vi "create_scan_steps.vi"(7 "number of steps":u32, 9 "step":i32, 10 "stop":i32, 11 "start":i32) -> (1 "array length":i32, 3 "single steps":i32[](array[numeric]))   [LabVIEW 2018]
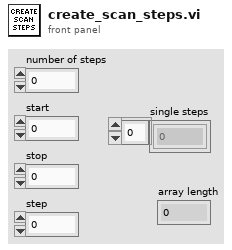
[diagram p1: front panel]
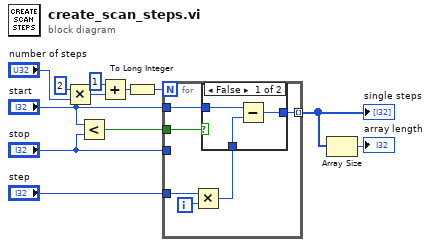
[diagram p0: block diagram]
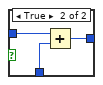
[diagram p2: hidden frame]
diagram:
  n1 = Multiply(x=u32 2, y="number of steps") -> (x*y=w8:u32)
  n2 = Less?(x="start", y="stop") -> (x < y?=w1:bool)
  n3 = Add(x=u32 1, y=w8) -> (x+y=w4:u32)
  n4 = To Long Integer(number=w4) -> (32bit integer=w9:i32)
  n5 = for {
    N: w9 -> [_]
    tunnel: "stop" -> [_]
    tunnel: "step" -> [w18]
    tunnel: [w14] -> w11 mode=indexing
    tunnel: "start" -> [w15]
    tunnel: w1 -> [w13]
    i -> [w17]
    n6 = Multiply(x=w18, y=w17) -> (x*y=w16:i32)
    n7 = case shown="False" w13 {
      tunnel: w16 -> [w19 w24]
      tunnel: w15 -> [w21 w23]
      tunnel: [w20 w22] -> w14
      frame False {
        n8 = Subtract(x=w21, y=w19) -> (x-y=w20:i32)
      }
      frame True {
        n9 = Add(x=w23, y=w24) -> (x+y=w22:i32)
      }
    }
  }
  "single steps" <- w11
  n10 = Array Size(array=w11) -> (size(s)=→"array length":i32)
